vi "icg_item_8.vi"() -> ()   [LabVIEW 2019]
uses:
  <vilib>/measure/NI_MAPro.lvlib
  <vilib>/measure/mamon.llb/Waveform Peak Detection for 1 Chan.vi
  <vilib>/Utility/file.llb/Read Delimited Spreadsheet (DBL).vi
panel:
  in  "Peak Threshold":dbl
  in  "Weight in kg":dbl
  in  "Height in cm":dbl
  out "Result of peak detection ( For Reference )":dbl[](graph)
  out "TLVE":dbl
  out "SV":dbl
  out "BMI":dbl
  out "ICG Graph":waveform(dbl)(graph)
  in  "file path (dialog if empty)":path
  # "ITEM 8"
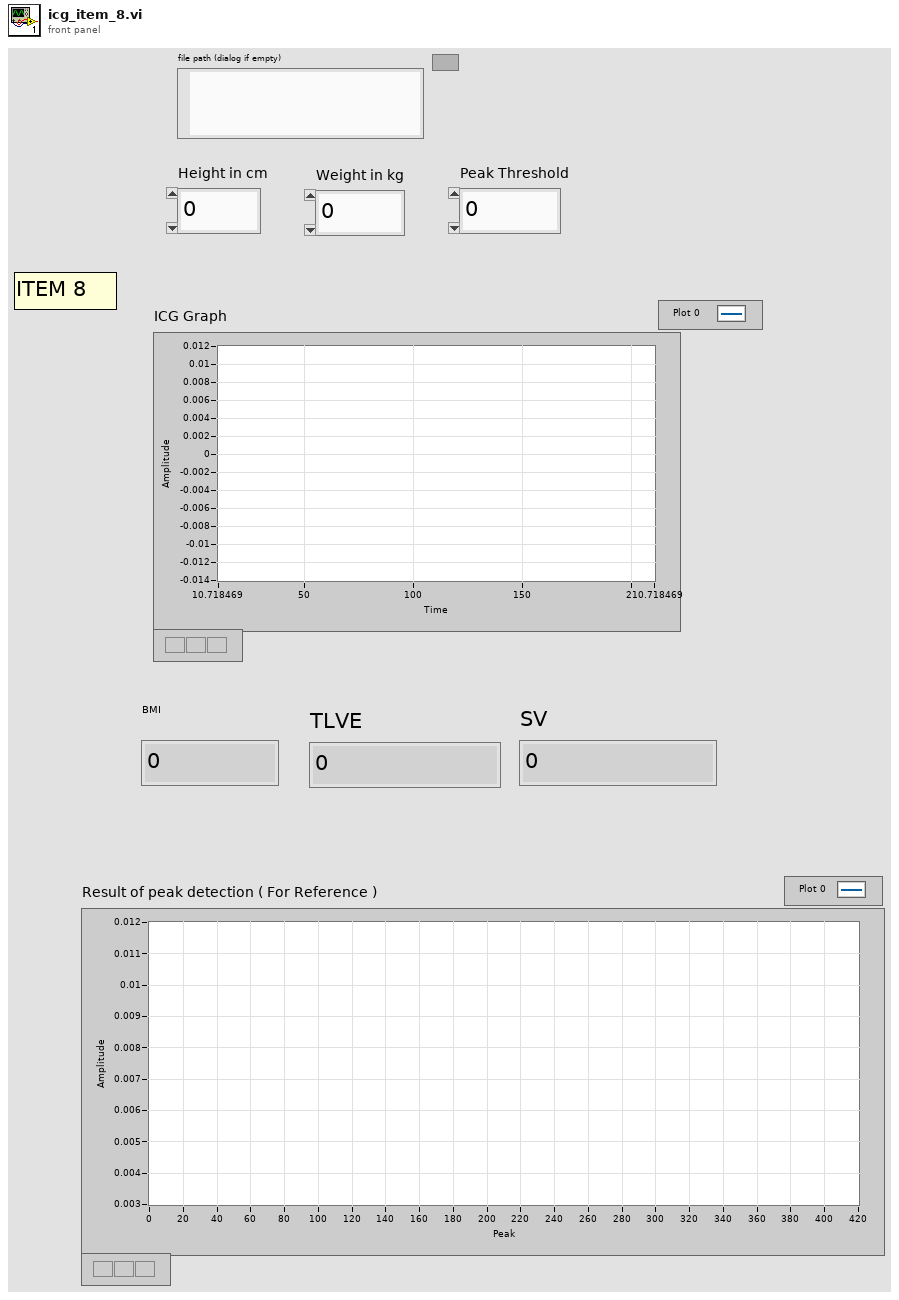
[diagram p1: front panel]
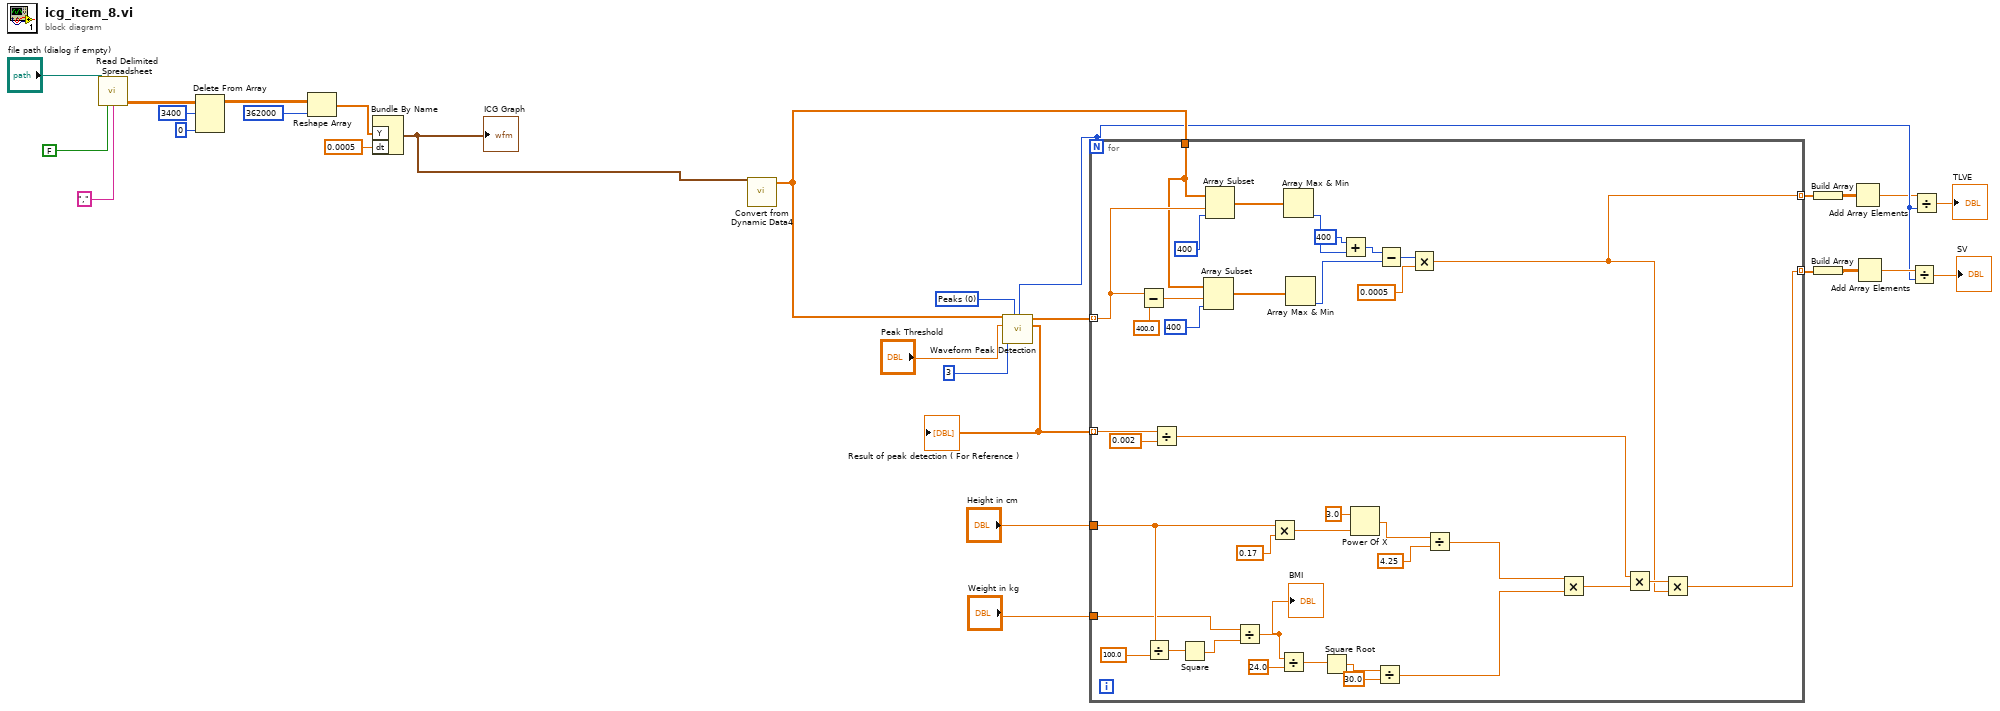
[diagram p0: block diagram]
diagram:
  w18 = u16 0 items=["Peaks", "Valleys"] ("peaks/valleys")
  n1 = call-poly <vilib>:"Read Delimited Spreadsheet.vi"("file path (dialog if empty)"="file path (dialog if empty)", "transpose? (F)"=FALSE, "delimiter (\\t)"="," ("delimiter (\\t)")) -> ("all rows"=w20:dbl[][])  [unwired: 7 in, 5 out]
  n2 = Delete From Array(array=w20, length=3400, index (row)=0 ("index")) -> (array with subset deleted=w19:dbl[][])  [unwired: 1 in, 1 out]
  n3 = Reshape Array(w19, 362000 ("dimension size")) -> (w24:dbl[])
  n4 = Bundle By Name("Y"=w24, "dt"=0.0005) -> (w6:waveform(dbl))  [unwired: 1 in]
  "ICG Graph" <- w6
  n5 = call "Convert from Dynamic Data4"("Dynamic Data Type"=w6) -> ("Array"=w15:dbl[])  [unwired: 3 in]
  n6 = call-poly <vilib>:"Waveform Peak Detection.vi"("peaks/valleys"=w18, "width"=3, "threshold"="Peak Threshold", "Signal In"=w15) -> ("Amplitudes"=w7:dbl[], "Locations"=w16:dbl[], "# found"=w10:i32)  [unwired: 3 in, 2 out]
  "Result of peak detection ( For Reference )" <- w7
  n7 = for {
    N: w10 -> [_]
    tunnel: w16 -> [w62] mode=indexing
    tunnel: w15 -> [w60]
    tunnel: [w32] -> w12 mode=indexing
    tunnel: w7 -> [w52] mode=indexing
    tunnel: [w31] -> w5 mode=indexing
    tunnel: "Height in cm" -> [w30]
    tunnel: "Weight in kg" -> [w29]
    n8 = Subtract(x=w62, y=400.0) -> (x-y=w65:dbl)
    n9 = Divide(x=w30, y=100.0) -> (x/y=w43:dbl)
    n10 = Divide(x=w52, y=0.002) -> (x/y=w33:dbl)
    n11 = Square(x=w43) -> (x^2=w44:dbl)
    n12 = Array Subset(array=w60, index=w65, length=400) -> (w59:dbl[])
    n13 = Array Subset(array=w60, index=w62, length=400) -> (w61:dbl[])
    n14 = Divide(x=w29, y=w44) -> (x/y=w50:dbl)
    "BMI" <- w50
    n15 = Multiply(x=w30, y=0.17) -> (x*y=w40:dbl)
    n16 = Divide(x=w50, y=24.0) -> (x/y=w46:dbl)
    n17 = Array Max & Min(array=w61) -> (min index (indices)=w55:i32)  [unwired: 3 out]
    n18 = Array Max & Min(array=w59) -> (min index (indices)=w58:i32)  [unwired: 3 out]
    n19 = Square Root(x=w46) -> (sqrt(x)=w47:dbl)
    n20 = Add(x=400, y=w55) -> (x+y=w53:i32)
    n21 = Power Of X(1:w40, 2:3.0 ("y")) -> (0:w41:dbl)
    n22 = Divide(x=w47, y=30.0) -> (x/y=w48:dbl)
    n23 = Subtract(x=w53, y=w58) -> (x-y=w57:i32)
    n24 = Multiply(x=w57, y=0.0005) -> (x*y=w31:dbl)
    n25 = Divide(x=w41, y=4.25) -> (x/y=w42:dbl)
    n26 = Multiply(x=w42, y=w48) -> (x*y=w45:dbl)
    n27 = Multiply(x=w33, y=w45) -> (x*y=w49:dbl)
    n28 = Multiply(x=w49, y=w31) -> (x*y=w32:dbl)
  }
  n29 = Build Array(w5) -> (w4:dbl[][])
  n30 = Build Array(w12) -> (w13:dbl[][])
  n31 = Add Array Elements(numeric array=w4) -> (sum=w9:dbl)
  n32 = Add Array Elements(numeric array=w13) -> (sum=w14:dbl)
  n33 = Divide(x=w14, y=w10) -> (x/y=→"SV":dbl)
  n34 = Divide(x=w9, y=w10) -> (x/y=→"TLVE":dbl)
